vi "AlignSubGroupOfControls.vi"(7 "Controls [t] / indicators [f]":bool, 8 "error in (no error)":errorcluster, 9 "Case structure contents to move away from":refnum<vi>[](array[refnum]), 10 "Controls to align and move":refnum<vi>[](array[refnum]), 11 "VI in":refnum<vi>) -> (0 "error out":errorcluster, 3 "VI ref (dup)":refnum<vi>)   [LabVIEW 2017, in "ErrorStructureDrawer.lvlib"]
doc: "Selects, and then aligns and moves, the specified controls, in order to move them away from the case structure which will be created around the specified items. The specified controls should all be controls, or all be indicators, and they will all be aligned together."
uses:
  ErrorStructureDrawer.lvlib
  <vilib>/Utility/miscctls.llb/LVDeltaXY32Cluster.ctl
  GetErrorIndicatorAlignTypeBD.vi
  GetErrorControlAlignTypeBD.vi
  GetErrorControlHorizSpacingBD.vi
  GetErrorIndicatorHorizSpacingBD.vi
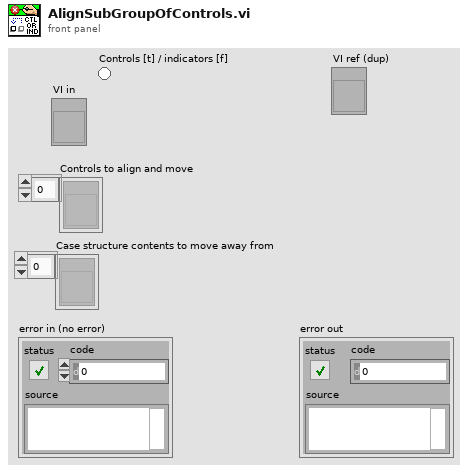
[diagram p1: front panel]
types:
  T1 = typedef "LVDeltaXY32Cluster.ctl" = cluster{"X":i32, "Y":i32}
  T2 = enum32{"Top Edges", "Vertical Centers", "Bottom Edges", "Left Edges", "Horizontal Centers", "Right Edges"}
  T3 = typedef "LVBoundsTypeDef.ctl" = cluster{"Width":u32, "Height":u32}
  T4 = typedef "LVPositionTypeDef.ctl" = cluster{"Left":i32, "Top":i32}
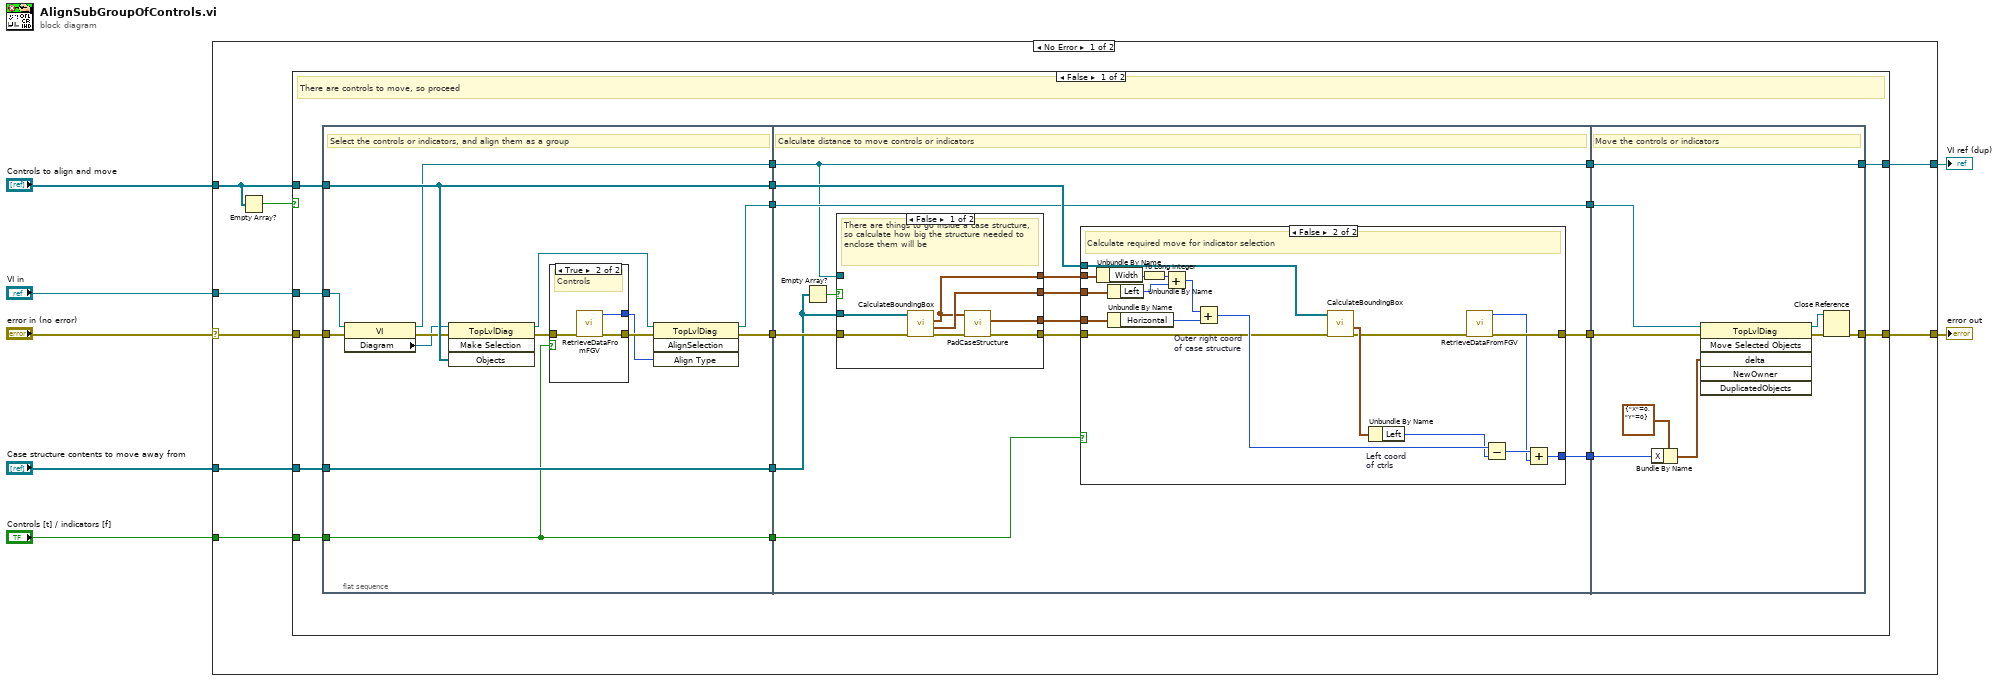
[diagram p0: block diagram]
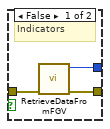
[diagram p2: hidden frame]
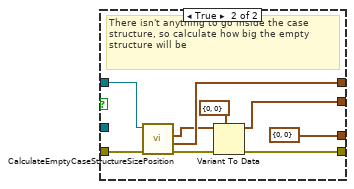
[diagram p3: hidden frame]
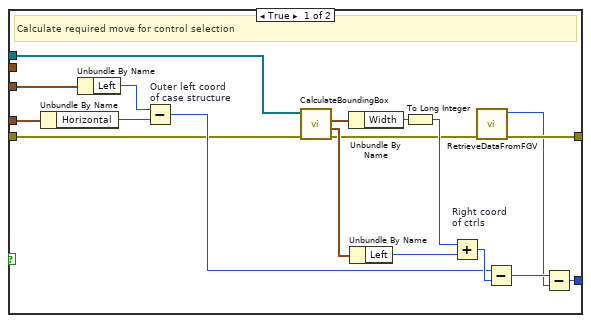
[diagram p4: hidden frame]
diagram:
  n1 = case shown="No Error" "error in (no error)" {
    selector: "error in (no error)" -> [w10 w130]
    tunnel: "Controls to align and move" -> [w9 _]
    tunnel: "Case structure contents to move away from" -> [w15 _]
    tunnel: "Controls [t] / indicators [f]" -> [w14 _]
    tunnel: [w13 w130] -> w4
    tunnel: "VI in" -> [w12 w129]
    tunnel: [w11 w129] -> w1
    frame No Error {
      n2 = Empty Array?(array=w9) -> (empty?=w8:bool)
      n3 = case shown="False" w8 {
        tunnel: w9 -> [w24 _]
        tunnel: w15 -> [w23 _]
        tunnel: w14 -> [w22 _]
        tunnel: [w21 w128] -> w11
        tunnel: [w20 w127] -> w13
        tunnel: w12 -> [w19 w128]
        tunnel: w10 -> [w16 w127]
        frame False {
          # "There are controls to move, so proceed"
          n4 = flat-sequence {
            tunnel: w22 -> [w41]
            tunnel: w23 -> [w46]
            tunnel: w24 -> [w45]
            tunnel: [w45] -> w32
            tunnel: [w46] -> w31
            tunnel: [w43] -> w30
            tunnel: [w41] -> w29
            tunnel: w19 -> [w35]
            tunnel: [w44] -> w28
            tunnel: [w34] -> w18
            tunnel: w16 -> [w33]
            tunnel: [w65] -> w27
            tunnel: [w63] -> w26
            tunnel: w32 -> [w64]
            tunnel: w31 -> [w55]
            tunnel: w30 -> [w60]
            tunnel: w29 -> [w57]
            tunnel: [w56] -> w25
            tunnel: w28 -> [w56]
            tunnel: w18 -> [w53]
            tunnel: [w53] -> w17
            tunnel: w27 -> [w123]
            tunnel: w26 -> [w124]
            tunnel: [w118] -> w21
            tunnel: [w119] -> w20
            tunnel: w25 -> [w122]
            tunnel: w17 -> [w118]
            frame #0 {
              # "Select the controls or indicators, and align them as a group"
              n5 = property class="VI"(reference=w35, error in=w33) -> (reference out=w34:refnum<vi>, error out=w37:errorcluster, "Diagram"=w36:refnum<vi>)
              n6 = invoke class="TopLvlDiag" method="Make Selection"(reference=w36, error in=w37, "Objects"=w45) -> (reference out=w42:refnum<vi>, error out=w38:errorcluster)  [unwired: 1 in, 2 out]
              n7 = case shown="True" w41 {
                tunnel: [w48 w52] -> w40
                tunnel: [w47 w51] -> w39
                tunnel: w38 -> [w49 w50]
                frame False {
                  # "Indicators"
                  n8 = call-poly "RetrieveDataFromFGV.vi"("error in (no error)"=w49) -> ("error out"=w48:errorcluster, "Indicators alignment type"=w47:T2)  [unwired: 9 in]
                }
                frame True {
                  # "Controls"
                  n9 = call-poly "RetrieveDataFromFGV.vi"("error in (no error)"=w50) -> ("error out"=w52:errorcluster, "Controls alignment type"=w51:T2)  [unwired: 9 in]
                }
              }
              n10 = invoke class="TopLvlDiag" method="AlignSelection"(reference=w42, error in=w40, "Align Type"=w39) -> (reference out=w44:refnum<vi>, error out=w43:errorcluster)  [unwired: 1 in, 2 out]
            }
            frame #1 {
              # "Calculate distance to move controls or indicators"
              n11 = Empty Array?(array=w55) -> (empty?=w54:bool)
              n12 = case shown="False" w54 {
                tunnel: [w72 w74] -> w62
                tunnel: [w71 cluster{"Horizontal":i32, "Vertical":i32} {"Horizontal"=0, "Vertical"=0} ("Offset for items from outer top left corner")] -> w61
                tunnel: w60 -> [w69 w81]
                tunnel: [w68 w75] -> w59
                tunnel: [w67 w78] -> w58
                tunnel: w55 -> [w66 _]
                tunnel: w53 -> [_ w80]
                frame False {
                  # "There are things to go inside a case structure, so calculate how big the structure needed to enclose them will be"
                  n13 = call "CalculateBoundingBox.vi"("error in (no error)"=w69, "Items"=w66) -> ("error out"=w70:errorcluster, "Current bounding box position"=w72:cluster{"Left":i32, "Top":i32}, "Size of bounding box for items"=w67:T3)  [unwired: 6 in, 1 out]
                  n14 = call "PadCaseStructure.vi"("error in (no error)"=w70, "Bounding box for items in"=w67) -> ("error out"=w68:errorcluster, "Offset for items from outer top left corner"=w71:cluster{"Horizontal":i32, "Vertical":i32})  [unwired: 7 in, 1 out]
                }
                frame True {
                  # "There isn't anything to go inside the case structure, so calculate how big the empty structure will be"
                  n15 = call "CalculateEmptyCaseStructureSizePosition.vi"("error in (no error)"=w81, "VI ref in"=w80) -> ("error out"=w77:errorcluster, "Case structure frame size"=w78:T3, "Case structure position"=w76:T4)  [unwired: 6 in, 1 out]
                  n16 = Variant To Data(error in=w77, type=cluster{"Left":i32, "Top":i32} {"Left"=0, "Top"=0} ("Current bounding box position"), Variant=w76) -> (data=w74:cluster{"Left":i32, "Top":i32}, error out=w75:errorcluster)
                }
              }
              n17 = case shown="False" w57 {
                tunnel: [w84 w102] -> w65
                tunnel: w64 -> [w99 w117]
                tunnel: [w93 w114] -> w63
                tunnel: w62 -> [w90 w113]
                tunnel: w61 -> [w89 w112]
                tunnel: w59 -> [w85 w109]
                tunnel: w58 -> [_ w108]
                frame True {
                  # "Calculate required move for control selection"
                  n18 = Unbundle By Name(w89) -> ("Horizontal"=w88:i32)
                  n19 = Unbundle By Name(w90) -> ("Left"=w87:i32)
                  n20 = Subtract "Outer left coord\nof case structure"(x=w87, y=w88) -> (x-y=w86:i32)
                  n21 = call "CalculateBoundingBox.vi"("error in (no error)"=w85, "Items"=w99) -> ("error out"=w83:errorcluster, "Current bounding box position"=w97:cluster{"Left":i32, "Top":i32}, "Size of bounding box for items"=w96:T3)  [unwired: 6 in, 1 out]
                  n22 = Unbundle By Name(w96) -> ("Width"=w92:u32)
                  n23 = Unbundle By Name(w97) -> ("Left"=w98:i32)
                  n24 = To Long Integer(number=w92) -> (32bit integer=w91:i32)
                  n25 = Add "Right coord\nof ctrls"(x=w91, y=w98) -> (x+y=w95:i32)
                  n26 = call-poly "RetrieveDataFromFGV.vi"("error in (no error)"=w83) -> ("error out"=w84:errorcluster, "Control terminals right-side whitespace (px)"=w82:i32)  [unwired: 9 in]
                  n27 = Subtract(x=w86, y=w95) -> (x-y=w94:i32)
                  n28 = Subtract(x=w94, y=w82) -> (x-y=w93:i32)
                }
                frame False {
                  # "Calculate required move for indicator selection"
                  n29 = Unbundle By Name(w108) -> ("Width"=w106:u32)
                  n30 = Unbundle By Name(w113) -> ("Left"=w107:i32)
                  n31 = Unbundle By Name(w112) -> ("Horizontal"=w111:i32)
                  n32 = To Long Integer(number=w106) -> (32bit integer=w105:i32)
                  n33 = Add(x=w105, y=w107) -> (x+y=w104:i32)
                  n34 = Add "Outer right coord\nof case structure"(x=w104, y=w111) -> (x+y=w110:i32)
                  n35 = call "CalculateBoundingBox.vi"("error in (no error)"=w109, "Items"=w117) -> ("error out"=w101:errorcluster, "Current bounding box position"=w116:cluster{"Left":i32, "Top":i32})  [unwired: 6 in, 2 out]
                  n36 = Unbundle By Name "Left coord\nof ctrls"(w116) -> ("Left"=w103:i32)
                  n37 = call-poly "RetrieveDataFromFGV.vi"("error in (no error)"=w101) -> ("error out"=w102:errorcluster, "Indicator terminals left-side whitespace (px)"=w100:i32)  [unwired: 9 in]
                  n38 = Subtract(x=w110, y=w103) -> (x-y=w115:i32)
                  n39 = Add(x=w115, y=w100) -> (x+y=w114:i32)
                }
              }
            }
            frame #2 {
              # "Move the controls or indicators"
              n40 = Bundle By Name(cluster=T1 {"X"=0, "Y"=0} ("X/Y Delta"), "X"=w124) -> (w126:T1)
              n41 = invoke class="TopLvlDiag" method="Move Selected Objects"(reference=w122, error in=w123, "delta"=w126) -> (reference out=w120:refnum<vi>, error out=w121:errorcluster)  [unwired: 3 in, 4 out]
              n42 = Close Reference(reference=w120, error in (no error)=w121) -> (error out=w119:errorcluster)
            }
          }
        }
        frame True {
          # "There are no controls to move - do nothing"
        }
      }
    }
    frame Error {
    }
  }
  "error out" <- w4
  "VI ref (dup)" <- w1
